vi "Volt Regulator.vi"(0 "InSpeed":dbl(slide) scale=0.0..22.0, 1 "Acceleration Thresh":cluster{dbl, dbl}(slide)={6.5, 8.85818181818182} scale=-10.0..10.0, 5 "Speed Threshold":dbl(slide)=6.5 scale=0.0..22.0, 7 "InACC":dbl(slide) scale=-10.0..10.0, 9 "Volt High Threshold":cluster{dbl, dbl}(slide)={6.5, 8.85818181818182} scale=0.0..14.0, 11 "InVoltage":dbl(slide) scale=0.0..14.0, 12 "ForceLow":bool=TRUE) -> (6 "NewGear":enum16{"High", "Low"}(ring)=enum."Low")   [LabVIEW 2014]
panel:
  in  "stop":bool
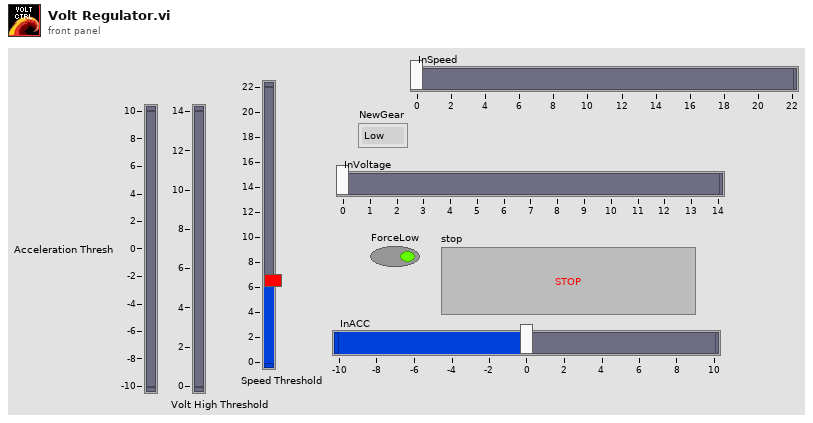
[diagram p1: front panel]
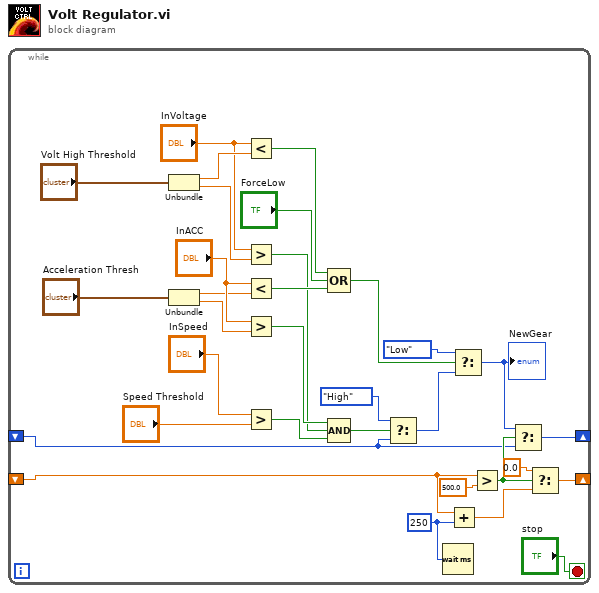
[diagram p0: block diagram]
diagram:
  n1 = while {
    shift-right: [w20] -> _
    shift-left: _ -> [w16]
    shift-right: [w24] -> _
    shift-left: _ -> [w15]
    stop <- "stop" stop-if-true
    w13 = u32 250 ("milliseconds to wait")
    n2 = Unbundle("Volt High Threshold") -> (w28:dbl, w27:dbl)
    n3 = Unbundle("Acceleration Thresh") -> (w10:dbl, w9:dbl)
    n4 = Less?(x="InVoltage", y=w28) -> (x < y?=w8:bool)
    n5 = Greater?(x="InVoltage", y=w27) -> (0:w2:bool)
    n6 = Less?(x="InACC", y=w10) -> (x < y?=w6:bool)
    n7 = Greater?(x="InACC", y=w9) -> (0:w3:bool)
    n8 = Greater?(x="InSpeed", y="Speed Threshold") -> (0:w1:bool)
    n9 = Compound Arithmetic op=OR(w8, "ForceLow", w6) -> (w5:bool)
    n10 = Compound Arithmetic op=AND(w3, w2, w1) -> (w4:bool)
    n11 = Select(t=enum16{"High", "Low"}."High", s=w4, f=w16) -> (s? t:f=w17:enum16{"High", "Low"})
    n12 = Wait (ms)(milliseconds to wait=w13) -> ()  [unwired: 1 out]
    n13 = Add(x=w15, y=w13) -> (x+y=w14:dbl)
    n14 = Select(t=enum16{"High", "Low"}."Low" ("Gear 2"), s=w5, f=w17) -> (s? t:f=w19:enum16{"High", "Low"})
    "NewGear" <- w19
    n15 = Greater?(x=w15, y=500.0) -> (0:w21:bool)
    n16 = Select(t=w19, s=w21, f=w16) -> (s? t:f=w20:enum16{"High", "Low"})
    n17 = Select(t=0.0, s=w21, f=w14) -> (s? t:f=w24:dbl)
  }
